vi "generate_input_line.vi"(9 "Size":i32=200, 10 "y":dbl) -> (0 "z Vector":dbl[](array[numeric]), 1 "Y Vector":dbl[](array[numeric]), 2 "X Vector":dbl[](array[numeric]))   [LabVIEW 2020, in "3DPC_SurfacePlot.xctl"]
uses:
  <vilib>/Native 3D Graph/xcontrol/3DPC_SurfacePlot.xctl
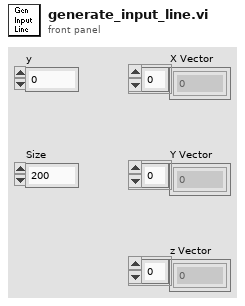
[diagram p1: front panel]
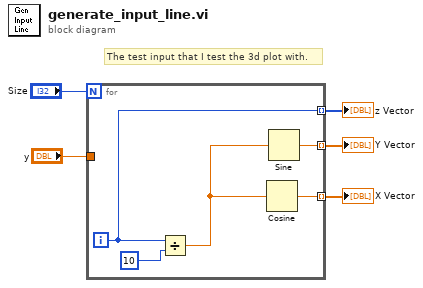
[diagram p0: block diagram]
diagram:
  # "The test input that I test the 3d plot with."
  n1 = for {
    N: "Size" -> [_]
    tunnel: [w8] -> w4 mode=indexing
    tunnel: [w7] -> w3 mode=indexing
    tunnel: [w6] -> w2 mode=indexing
    tunnel: "y" -> [_]
    i -> [w6]
    n2 = Divide(x=w6, y=10) -> (x/y=w9:dbl)
    n3 = Cosine(x=w9) -> (cos(x)=w7:dbl)
    n4 = Sine(x=w9) -> (sin(x)=w8:dbl)
  }
  "z Vector" <- w2
  "Y Vector" <- w4
  "X Vector" <- w3
